vi "Factorial using While loop.vi"() -> ()   [LabVIEW 2020]
panel:
  out "current time":timestamp
  out "Factorial of Input N using for loop":i32
  in  "Input N":i32
  out "Factorial of Input N using while loop":i32
  in  "Input N":i32
  # "1-a)"
  # "1-b)"
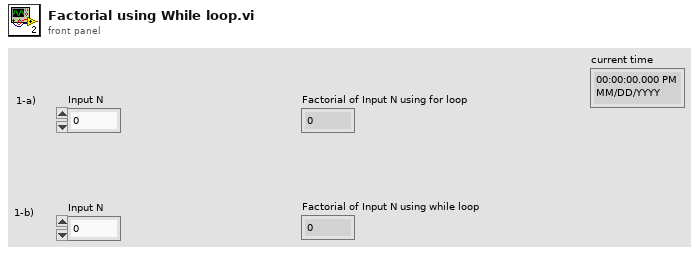
[diagram p1: front panel]
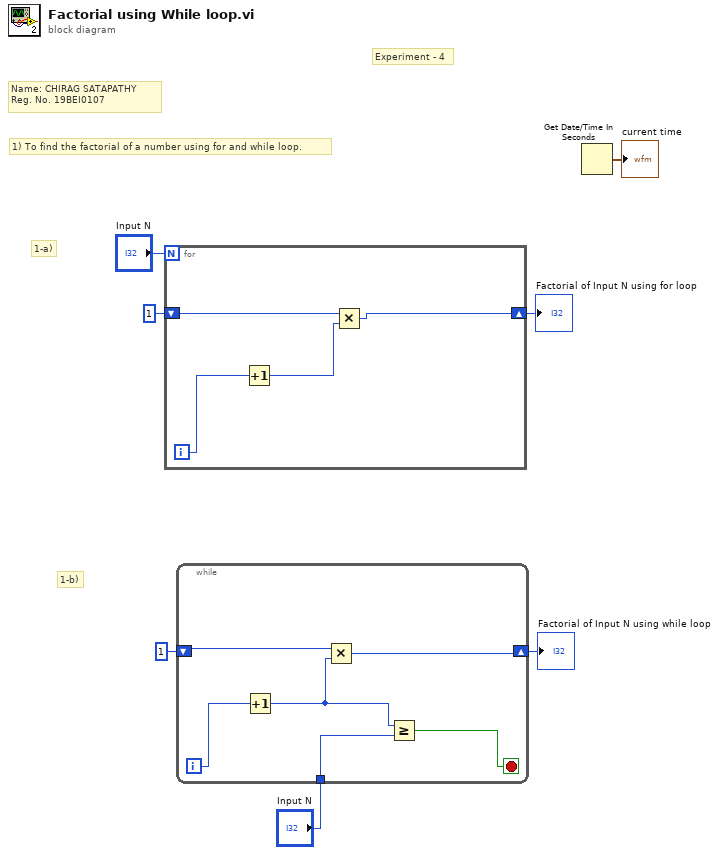
[diagram p0: block diagram]
diagram:
  # "Experiment - 4"
  # "1-b)"
  # "1-a)"
  # "Name: CHIRAG SATAPATHY\nReg. No. 19BEI0107"
  # "1) To find the factorial of a number using for and while loop."
  n1 = for {
    N: "Input N" -> [_]
    shift-right: [w10] -> w2
    shift-left: 1 -> [w9]
    i -> [w11]
    n2 = Increment(x=w11) -> (x+1=w8:i32)
    n3 = Multiply(x=w9, y=w8) -> (x*y=w10:i32)
  }
  "Factorial of Input N using for loop" <- w2
  n4 = while {
    tunnel: "Input N" -> [w16]
    shift-right: [w14] -> w5
    shift-left: 1 -> [w15]
    i -> [w17]
    stop <- w12 stop-if-true
    n5 = Increment(x=w17) -> (x+1=w13:i32)
    n6 = Multiply(x=w15, y=w13) -> (x*y=w14:i32)
    n7 = Greater Or Equal?(x=w13, y=w16) -> (x >= y?=w12:bool)
  }
  "Factorial of Input N using while loop" <- w5
  n8 = Get Date/Time In Seconds() -> (seconds since 1Jan1904=→"current time":timestamp)
